vi "5) Using Waveform Chart (Temperature Conversion).vi"() -> ()   [LabVIEW 2018]
panel:
  in  "milliseconds to wait":u32
  in  "Stop":bool
  out "Waveform Graph":dbl[](graph)
  out "Temperature (C)":dbl
  out "Waveform Chart":dbl(graph)
  in  "Switch":bool
  in  "Temperature (F)":dbl(slide) scale=0.0..100.0
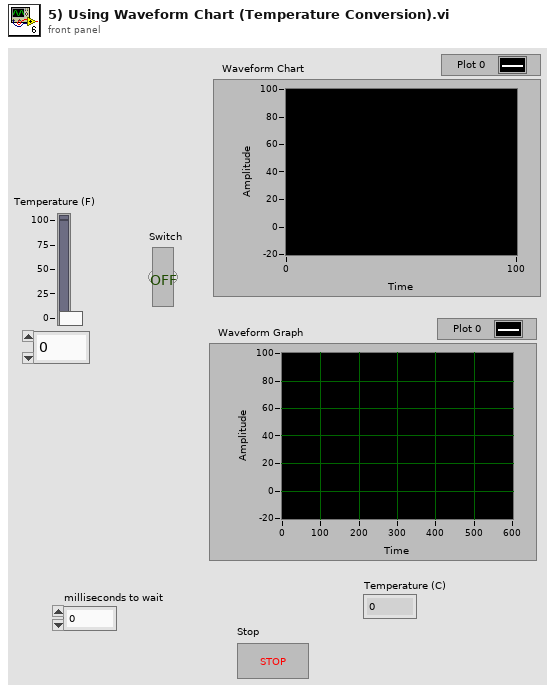
[diagram p1: front panel]
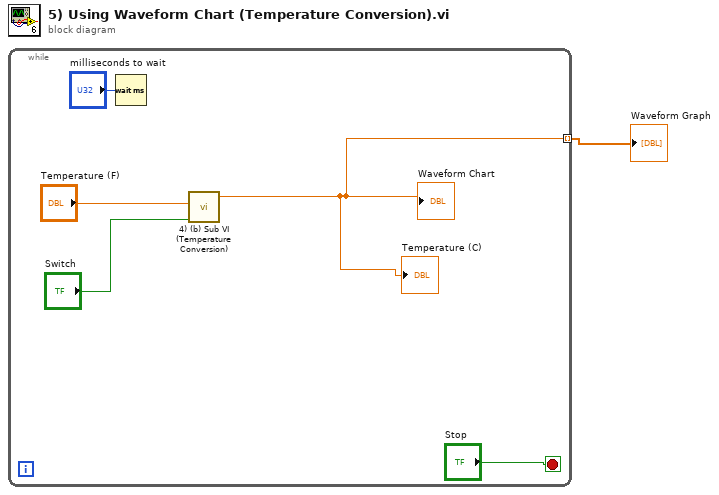
[diagram p0: block diagram]
diagram:
  n1 = while {
    tunnel: [w3] -> w1 mode=indexing
    stop <- "Stop" stop-if-true
    n2 = Wait (ms)(milliseconds to wait="milliseconds to wait") -> ()  [unwired: 1 out]
    n3 = call "4) (b) Sub VI (Temperature Conversion).vi"("Boolean"="Switch", "Temperature (F)"="Temperature (F)") -> ("Numeric"=w3:dbl)  [unwired: 9 in]
    "Waveform Chart" <- w3
    "Temperature (C)" <- w3
  }
  "Waveform Graph" <- w1
